vi "Alternate BG Color.vi"(6 "Row or Col Option":T1, 8 "错误输入":errorcluster, 9 "Second BG Color":u32(colorbox), 10 "First BG Color":u32(colorbox), 11 "Table Ref In":refnum<vi>) -> (0 "错误输出":errorcluster, 3 "Table Ref Out":refnum<vi>)   [LabVIEW 2012, in "Table Tool.lvlib"]
uses:
  Table Tool.lvlib
  Custum Type/Selet Row or Col.ctl
  Custum Type/GetOrSet.ctl
  Property/Set Or Get Num of Rows or Cols.vi
  Property/Set Or get ActiveCell Bk Color.vi
  Property/Set  ActiveCell by Row Or Column.vi
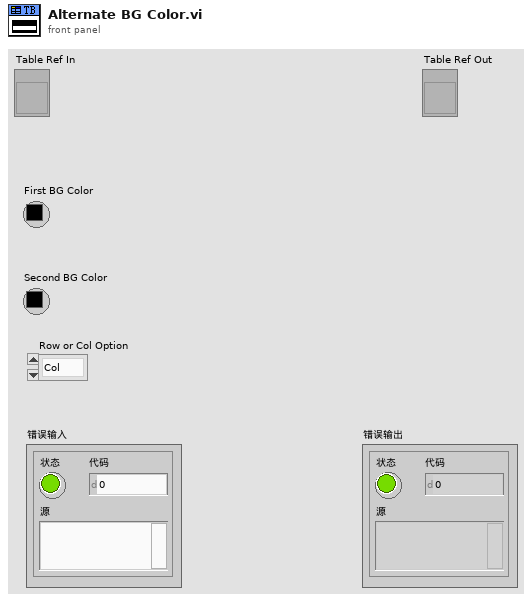
[diagram p1: front panel]
types:
  T1 = typedef "Table Tool.lvlib/Selet Row or Col.ctl" = enum16{"Col", "Row"}
  T2 = typedef "Table Tool.lvlib/GetOrSet.ctl" = enum16{"Get", "Set"}
  T3 = enum16{"All Rows and Cols", "Row Head", "Col Head", "N Row", "N Col"}
  T4 = typedef "LVRowAndColumnTypeDef.ctl" = cluster{"Row":i32, "Column":i32}
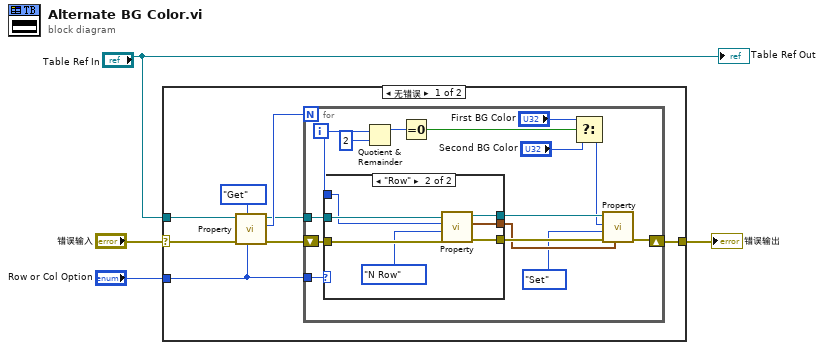
[diagram p0: block diagram]
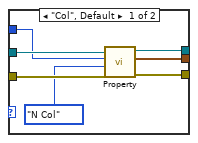
[diagram p2: hidden frame]
diagram:
  n1 = case shown="无错误" "错误输入" {
    selector: "错误输入" -> [w12 w42]
    tunnel: [w5 w42] -> w3
    tunnel: "Row or Col Option" -> [w8 _]
    tunnel: "Table Ref In" -> [w11 _]
    frame No Error {
      n2 = call-poly "Property.vi"("Row or Col Option"=w8, "Mode"=GetOrSet."Get", "error in (no error)"=w12, "Table Ref In"=w11) -> ("error out"=w6:errorcluster, "Number of Rows or Cols Out"=w9:u32, "Table Ref Out"=w7:refnum<vi>)  [unwired: 5 in]
      n3 = for {
        N: w9 -> [_]
        tunnel: w8 -> [w23]
        tunnel: w7 -> [w27]
        shift-right: [w13] -> w5
        shift-left: w6 -> [w25]
        i -> [w21]
        n4 = case shown="\"Row\"" w23 {
          tunnel: w27 -> [w31 w41]
          tunnel: [w34 w40] -> w26
          tunnel: w25 -> [w30 w39]
          tunnel: [w33 w38] -> w24
          tunnel: w21 -> [w29 w36]
          tunnel: [w32 w35] -> w22
          frame "Col", Default {
            n5 = call-poly "Property.vi"("error in (no error)"=w30, "Option"=T3."N Col", "N"=w29, "Table Ref In"=w31) -> ("error out"=w33:errorcluster, "ActiveCell Out"=w32:T4, "Table Ref Out"=w34:refnum<vi>)  [unwired: 5 in]
          }
          frame "Row" {
            n6 = call-poly "Property.vi"("error in (no error)"=w39, "Option"=T3."N Row", "N"=w36, "Table Ref In"=w41) -> ("error out"=w38:errorcluster, "ActiveCell Out"=w35:T4, "Table Ref Out"=w40:refnum<vi>)  [unwired: 5 in]
          }
        }
        n7 = Quotient & Remainder(x=w21, y=2) -> (x-y*floor(x/y)=w19:i32)  [unwired: 1 out]
        n8 = Equal To 0?(x=w19) -> (x = 0?=w16:bool)
        n9 = Select(t="First BG Color", s=w16, f="Second BG Color") -> (s? t:f=w15:u32)
        n10 = call-poly "Property.vi"("Active Cell"=w22, "error in (no error)"=w24, "Mode"=GetOrSet."Set", "BK Color In"=w15, "Table Ref In"=w26) -> ("error out"=w13:errorcluster)  [unwired: 4 in, 2 out]
      }
    }
    frame Error {
    }
  }
  "错误输出" <- w3
  "Table Ref Out" <- "Table Ref In"
